vi "Condiciones_Cambios e intervalos entre velocidades_usando strings.vi"() -> ()   [LabVIEW 2013]
panel:
  out "AlarmaTemp":bool
  out "Temperatura":dbl(slide) scale=0.0..100.0
  out "Cambio":string
  out "Cuarta":bool
  out "Segunda":bool
  out "Tercera":bool
  out "Primera":bool
  out "velocidad":i32(knob) scale=0.0..180.0
  # "Si la temperatura es mayor a 75 y la velocidad es mayor a 120 encender alarma de calentamiento"
  # "Elaborar un programa donde se genere la velocidad entre 1-180,\nluego de acuerdo a la velocidad que se alcance en que cambio se \nencuentra y escribir en el string indicator el cambio\n\n1-40 primera\n41-60 segunda\n61-80 tercera\n81-180 cuarta"
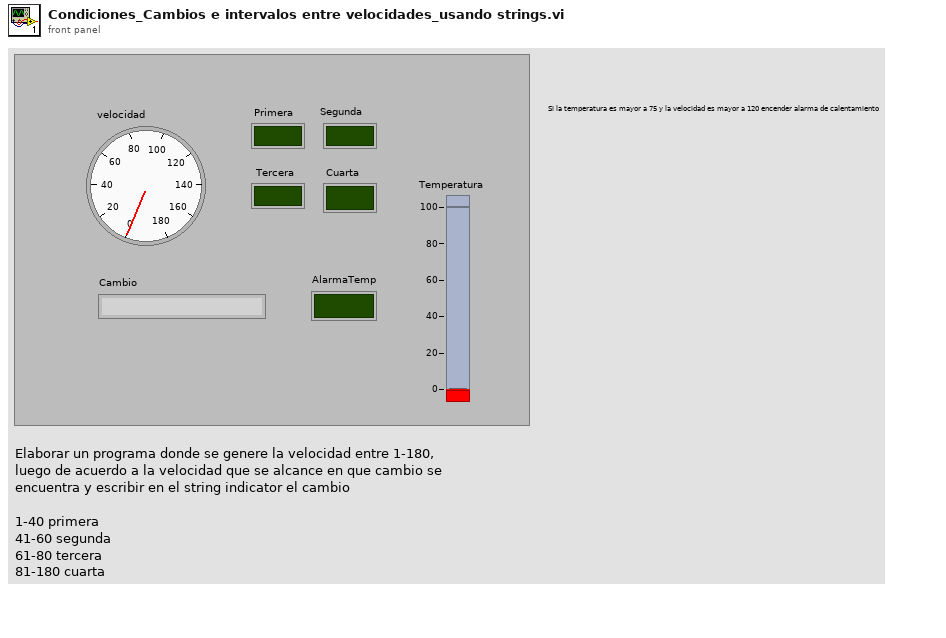
[diagram p1: front panel]
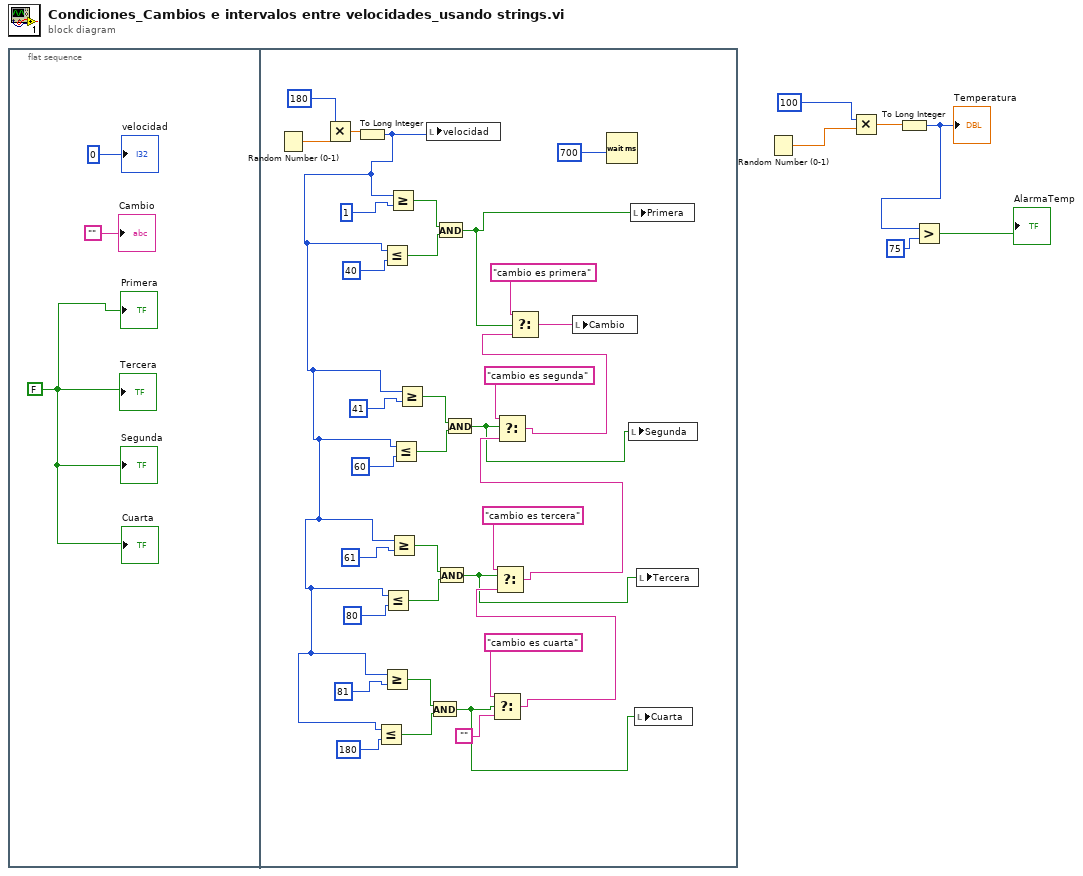
[diagram p0: block diagram]
diagram:
  n1 = flat-sequence {
    frame #0 {
      w7 = FALSE
      "velocidad" <- 0
      "Primera" <- w7
      "Tercera" <- w7
      "Segunda" <- w7
      "Cuarta" <- w7
      "Cambio" <- ""
    }
    frame #1 {
      n2 = Random Number (0-1)() -> (number: 0 to 1=w42:dbl)
      n3 = Multiply(x=180, y=w42) -> (x*y=w41:dbl)
      n4 = To Long Integer(number=w41) -> (32bit integer=w17:i32)
      n5 = Less Or Equal?(x=w17, y=180) -> (x <= y?=w21:bool)
      n6 = Less Or Equal?(x=w17, y=40) -> (x <= y?=w37:bool)
      n7 = Greater Or Equal?(x=w17, y=81) -> (x >= y?=w20:bool)
      n8 = Less Or Equal?(x=w17, y=80) -> (x <= y?=w24:bool)
      n9 = Greater Or Equal?(x=w17, y=1) -> (x >= y?=w38:bool)
      n10 = Greater Or Equal?(x=w17, y=61) -> (x >= y?=w25:bool)
      n11 = Less Or Equal?(x=w17, y=60) -> (x <= y?=w33:bool)
      n12 = Greater Or Equal?(x=w17, y=41) -> (x >= y?=w32:bool)
      n13 = local write "velocidad"(w17) -> ()
      n14 = And(x=w20, y=w21) -> (x .and. y?=w11:bool)
      n15 = And(x=w38, y=w37) -> (x .and. y?=w35:bool)
      n16 = And(x=w25, y=w24) -> (x .and. y?=w12:bool)
      n17 = And(x=w32, y=w33) -> (x .and. y?=w13:bool)
      n18 = Select(t="cambio es cuarta", s=w11, f="") -> (s? t:f=w15:string)
      n19 = Select(t="cambio es tercera", s=w12, f=w15) -> (s? t:f=w22:string)
      n20 = Select(t="cambio es segunda", s=w13, f=w22) -> (s? t:f=w28:string)
      n21 = Select(t="cambio es primera", s=w35, f=w28) -> (s? t:f=w34:string)
      n22 = local write "Cambio"(w34) -> ()
      n23 = Wait (ms)(milliseconds to wait=u32 700 ("millisecond timer value")) -> ()  [unwired: 1 out]
      n24 = local write "Segunda"(w13) -> ()
      n25 = local write "Primera"(w35) -> ()
      n26 = local write "Cuarta"(w11) -> ()
      n27 = local write "Tercera"(w12) -> ()
    }
  }
  n28 = Random Number (0-1)() -> (number: 0 to 1=w5:dbl)
  n29 = Multiply(x=100, y=w5) -> (x*y=w4:dbl)
  n30 = To Long Integer(number=w4) -> (32bit integer=w3:i32)
  "Temperatura" <- w3
  n31 = Greater?(x=w3, y=75) -> (0:→"AlarmaTemp":bool)
